vi "Serial Write.vi"(8 "error in (no error)":errorcluster, 10 "write buffer":string, 11 "VISA resource name":refnum<visa-resource-name>) -> (0 "error out":errorcluster, 1 "Pass?":bool, 2 "return count":u32, 3 "VISA resource name out":refnum<visa-resource-name>)   [LabVIEW 2025, in "SerialPort.lvlib"]
uses:
  <vilib>/Serial Port/SerialPort.lvlib
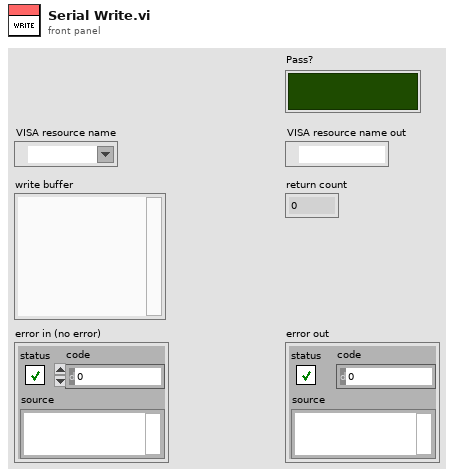
[diagram p1: front panel]
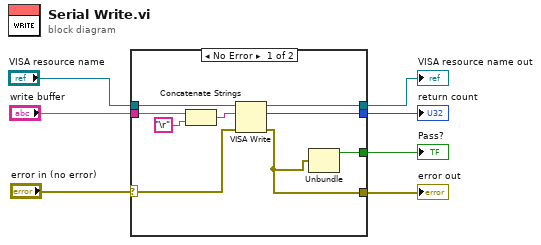
[diagram p0: block diagram]
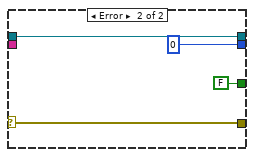
[diagram p2: hidden frame]
diagram:
  n1 = case shown="No Error" "error in (no error)" {
    selector: "error in (no error)" -> [w12 w18]
    tunnel: [w16 u32 0 ("return count")] -> w7
    tunnel: [w9 w18] -> w6
    tunnel: "write buffer" -> [w15 _]
    tunnel: "VISA resource name" -> [w14 w20]
    tunnel: [w13 w20] -> w3
    tunnel: [w8 FALSE ("status")] -> w1
    frame No Error {
      n2 = Concatenate Strings(w15, "\r") -> (w11:string)
      n3 = VISA Write(VISA resource name=w14, write buffer=w11, error in (no error)=w12) -> (VISA resource name out=w13:refnum<visa-resource-name>, return count=w16:u32, error out=w9:errorcluster)
      n4 = Unbundle(w9) -> ("status"=w8:bool)  [unwired: 2 out]
    }
    frame Error {
    }
  }
  "return count" <- w7
  "error out" <- w6
  "VISA resource name out" <- w3
  "Pass?" <- w1
